vi "Post Source Distribution.vi"(5 "Files Generated by Build":path[](array[path]), 6 "Top Level/Always Included VIs":path[](array[path]), 7 "Destination Path":path, 8 "error in (no error)":errorcluster, 9 "Target Name":string, 10 "Build Specification Name":string, 11 "Project Path":path) -> (0 "error out":errorcluster)   [LabVIEW 2020]
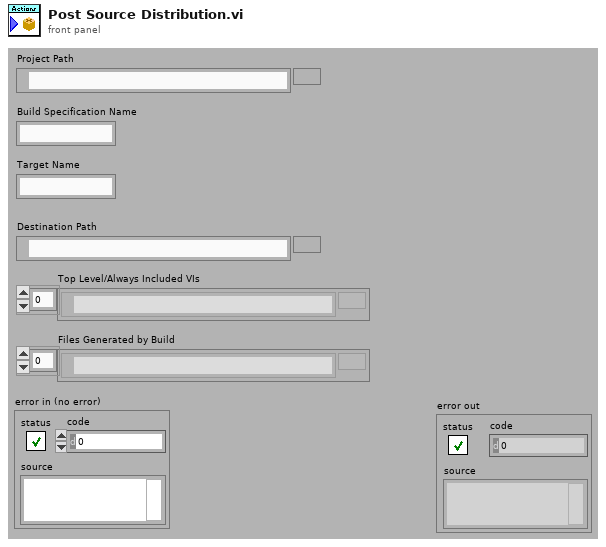
[diagram p1: front panel]
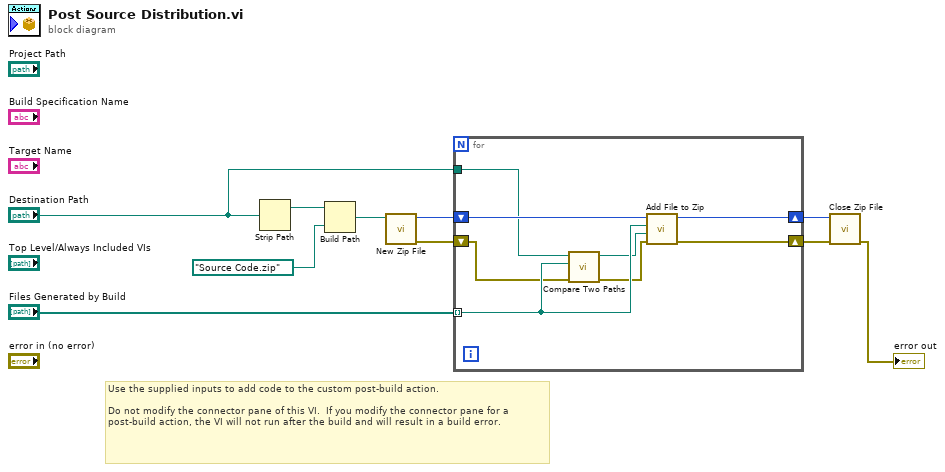
[diagram p0: block diagram]
diagram:
  # "Use the supplied inputs to add code to the custom post-build action.\n\nDo not modify the connector pane of this VI.  If you modify the connector pane for a post-build action, the VI will not run after the build and will result in a build error."
  n1 = Strip Path(path="Destination Path") -> (stripped path=w10:path)  [unwired: 1 out]
  n2 = Build Path(base path=w10, name or relative path=path "Source Code.zip") -> (appended path=w8:path)
  n3 = call <vilib>:"New Zip File.vi"("target"=w8) -> ("error out"=w7:errorcluster, "zip file out"=w6:i64)  [unwired: 4 in, 1 out]
  n4 = for {
    shift-right: [w17] -> w5
    shift-left: w7 -> [w12]
    shift-right: [w16] -> w4
    shift-left: w6 -> [w18]
    tunnel: "Files Generated by Build" -> [w14] mode=indexing
    tunnel: "Destination Path" -> [w15]
    n5 = call <vilib>:"Compare Two Paths.vi"("error in (no error)"=w12, "Path 2"=w14, "Path 1"=w15) -> ("error out"=w11:errorcluster, "Relative Path from 1 to 2"=w13:path)  [unwired: 5 in, 2 out]
    n6 = call <vilib>:"Add File to Zip.vi"("error in (no error)"=w11, "destination path in zip"=w13, "source file path"=w14, "zip file in"=w18) -> ("error out"=w17:errorcluster, "zip file out"=w16:i64)  [unwired: 6 in]
  }
  n7 = call <vilib>:"Close Zip File.vi"("error in (no error)"=w5, "zip file in"=w4) -> ("error out"=→"error out":errorcluster)  [unwired: 5 in]
